vi "Set Case Sensitive.vi"(8 "error in (no error)":errorcluster, 10 "Case Sensitive Suggestions?":bool, 11 "IntelliSense String in":refnum<class "IntelliSenseStringControl.lvclass">) -> (0 "error out":errorcluster, 3 "IntelliSense String out":refnum<class "IntelliSenseStringControl.lvclass">)   [LabVIEW 2016, in "StringIntelliSense.lvlib" / "IntelliSenseStringControl.lvclass"]
uses:
  IntelliSenseStringControl.lvclass
  IntelliSenseStringControl.lvclass/IntelliSenseStringControl.ctl
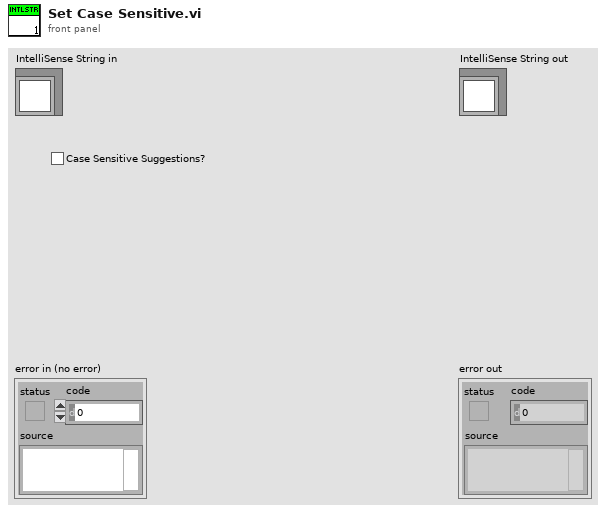
[diagram p1: front panel]
types:
  T1 = typedef "StringIntelliSense.lvlib/IntelliSenseStringControl.lvclass/String Monitor Details.ctl" = cluster{"Str ctrl Suggestion":string[], "Case Sensitive Suggestions?":bool, "Append User String to Suggestion?":bool, "Autofill Suggestion Choices?":bool}
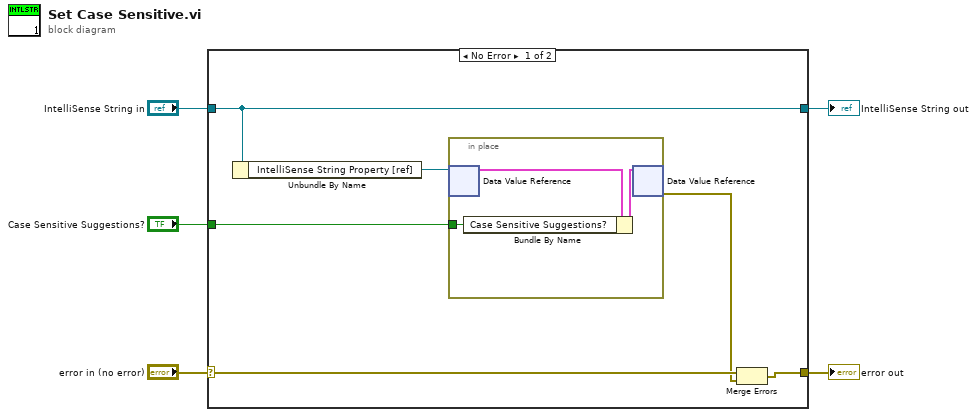
[diagram p0: block diagram]
diagram:
  n1 = case shown="No Error" "error in (no error)" {
    selector: "error in (no error)" -> [w11 w16]
    tunnel: [w7 w16] -> w4
    tunnel: [w10 w15] -> w2
    tunnel: "IntelliSense String in" -> [w10 w15]
    tunnel: "Case Sensitive Suggestions?" -> [w8 _]
    frame No Error {
      n2 = Unbundle By Name(w10) -> ("IntelliSense String Property [ref]"=w9:refnum<data-value>)
      n3 = in-place {
        in-place-border: w8 -> [w13]
        n4 = in-place-dvr #1(w9) -> (w14:T1)  [unwired: 1 out]
        n5 = Bundle By Name(cluster=w14, "Case Sensitive Suggestions?"=w13) -> (w12:T1)
        n6 = in-place-dvr #1(w12) -> (w6:errorcluster)  [unwired: 1 out]
      }
      n7 = Merge Errors(w11, w6) -> (w7:errorcluster)
    }
    frame Error {
    }
  }
  "error out" <- w4
  "IntelliSense String out" <- w2
